vi "UIRef.vi"(8 "error in":errorcluster, 11 "SQLite editor node in":refnum<class "SQLite editor node.lvclass">) -> (0 "error out":errorcluster, 2 "VI refnum":refnum<vi>, 3 "SQLite editor node out":refnum<class "SQLite editor node.lvclass">)   [LabVIEW 2014, in "SQLite editor node.lvclass"]
doc: "Returns a reference to the main UI VI to display in the configuration editor. This VI can be used to programmatically select which UI to display, or can be hard-coded to a single VI."
uses:
  SQLite editor node.lvclass
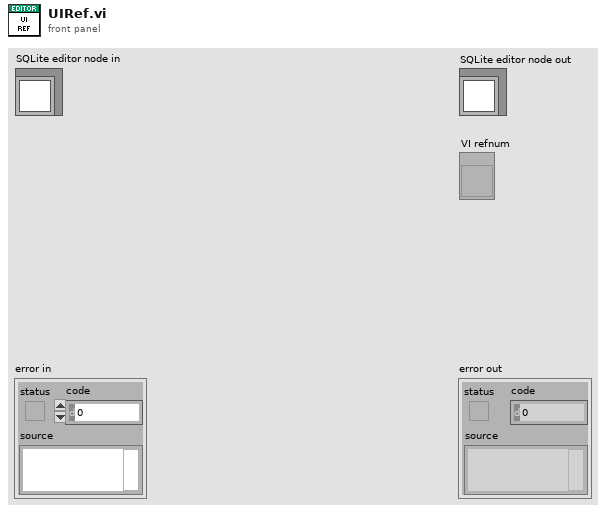
[diagram p1: front panel]
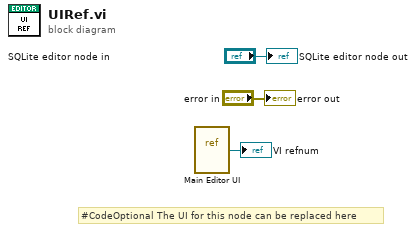
[diagram p0: block diagram]
diagram:
  # "#CodeOptional The UI for this node can be replaced here"
  n1 = vi-ref "Main Editor UI.vi"() -> (→"VI refnum":refnum<vi>)
  "error out" <- "error in"
  "SQLite editor node out" <- "SQLite editor node in"
